vi "Device Properties - Get Timeout.vi"(8 "error in (no error)":errorcluster, 11 "Device Ref in":T1 format="%.0x") -> (0 "error out":errorcluster, 2 "IP Address":i32, 3 "Device Ref out":T1 format="%.0x")   [LabVIEW 2012, in "Shared Variable Custom Device.lvlib"]
doc: "Gets the IP Address of the custom device target."
uses:
  Shared Variable Custom Device.lvlib
  <vilib>/NI Veristand/Custom Device API/Custom Device Item Ref.ctl
  Shared Variable Globals.vi
  <vilib>/NI Veristand/Custom Device API/Get Item Property (I32).vi
  <vilib>/NI Veristand/Custom Device API/Custom Device API.lvlib
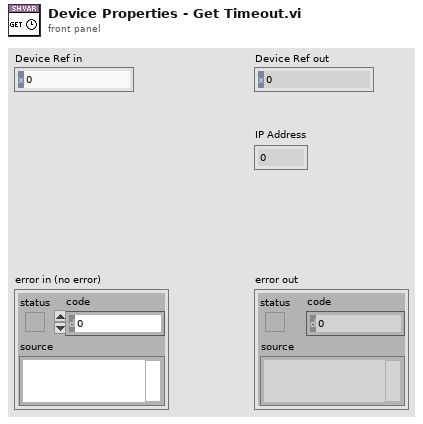
[diagram p1: front panel]
types:
  T1 = typedef "Custom Device API.lvlib/Custom Device Item Ref.ctl" = u64
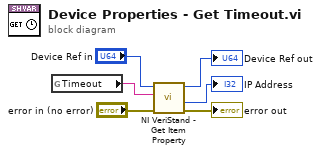
[diagram p0: block diagram]
diagram:
  n1 = global read "Shared Variable Globals.vi" "Timeout"() -> (w6:string)
  n2 = call-poly <vilib>:"NI VeriStand - Get Item Property.vi"("error in (no error)"="error in (no error)", "Property Name"=w6, "Item Ref in"="Device Ref in") -> ("error out"=→"error out":errorcluster, "Value"=→"IP Address":i32, "Item Ref out"=→"Device Ref out":T1)  [unwired: 5 in, 1 out]
